vi "SaveQueueCreate.vi"(2 "error in (no error)":errorcluster) -> (0 "error out":errorcluster, 1 "Save queue":refnum<queue>)   [LabVIEW 2017]
uses:
  SaveQueueCluster.ctl
  SaveMessage.ctl
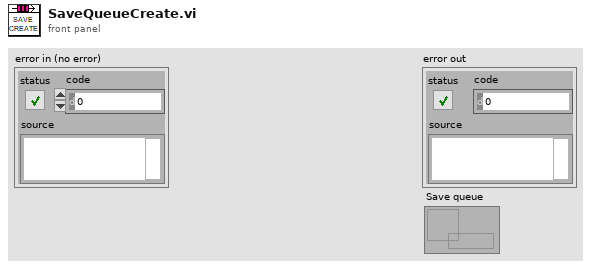
[diagram p1: front panel]
types:
  T1 = typedef "SaveQueueCluster.ctl" = cluster{"Save message":T2, "NumericValue":dbl, "String":string}
  T2 = typedef "SaveMessage.ctl" = enum16{"StartSaving", "StopSaving", "Ch1Value", "Ch2Value", "Ch3Value", "Error", "WriteFile", "Halt"}
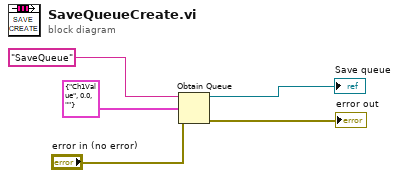
[diagram p0: block diagram]
diagram:
  n1 = Obtain Queue(name (unnamed)="SaveQueue", element data type=T1 {"Save message"=enum."Ch1Value", "NumericValue"=0.0, "String"=""} ("SaveQueueCluster"), error in (no error)="error in (no error)") -> (queue out=→"Save queue":refnum<queue>, error out=→"error out":errorcluster)  [unwired: 2 in, 1 out]
